vi "Comm String Flush Port.vi"(0 "niDTS Comm String in":refnum<class "niDTS Comm String.lvclass">, 7 "Read Data (F)":bool, 9 "Log Data (F)":bool, 11 "error in (no error)":errorcluster) -> (4 "niDTS Comm String out":refnum<class "niDTS Comm String.lvclass">, 8 "Read Data":string, 15 "error out":errorcluster)   [LabVIEW 2015, in "niDTS CommLib.lvlib" / "niDTS Comm String.lvclass"]
uses:
  niDTS Comm String.lvclass
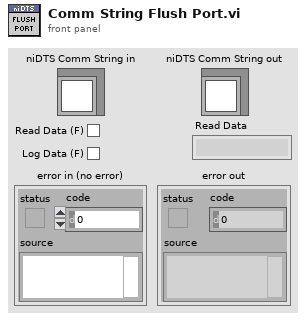
[diagram p1: front panel]
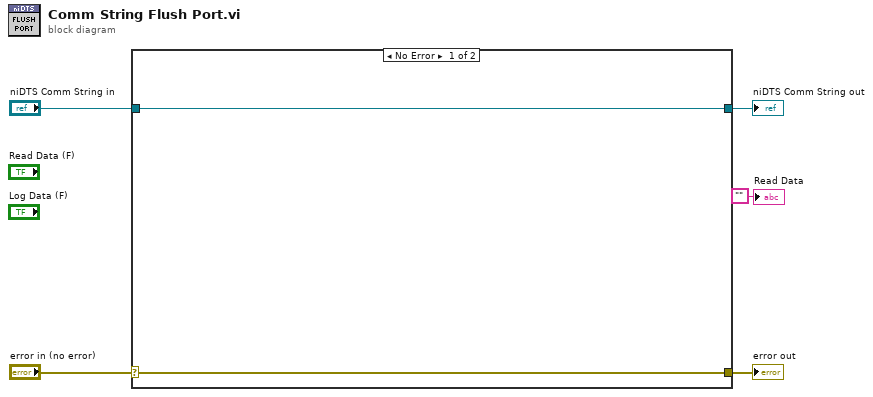
[diagram p0: block diagram]
diagram:
  n1 = case shown="No Error" "error in (no error)" {
    selector: "error in (no error)" -> [w6 w9]
    tunnel: [w6 w9] -> w4
    tunnel: [w7 w8] -> w2
    tunnel: "niDTS Comm String in" -> [w7 w8]
    frame No Error {
    }
    frame Error {
    }
  }
  "error out" <- w4
  "niDTS Comm String out" <- w2
  "Read Data" <- ""
